vi "QueryWavelength.vi"(8 "error in (no error)":errorcluster, 11 "HRS_Spectrometer in":refnum<class "HRS_Spectrometer.lvclass">) -> (0 "error out":errorcluster, 3 "HRS_Spectrometer out":refnum<class "HRS_Spectrometer.lvclass">)   [LabVIEW 2023, in "HRS_Spectrometer.lvlib" / "HRS_Spectrometer.lvclass"]
uses:
  HRS_Spectrometer.lvclass
  HRS_Spectrometer.lvclass/HRS_Spectrometer.ctl
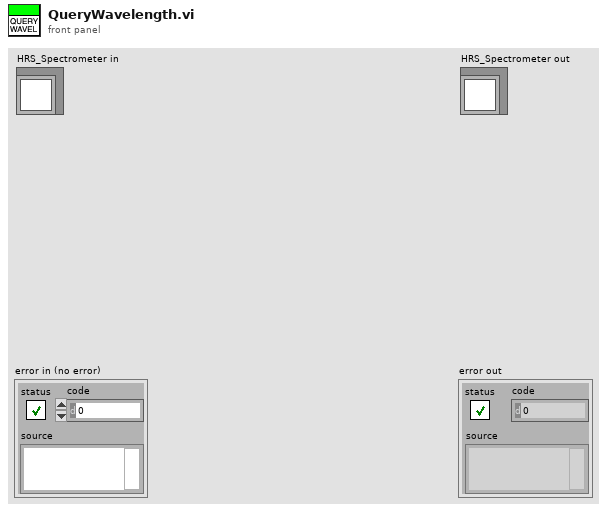
[diagram p1: front panel]
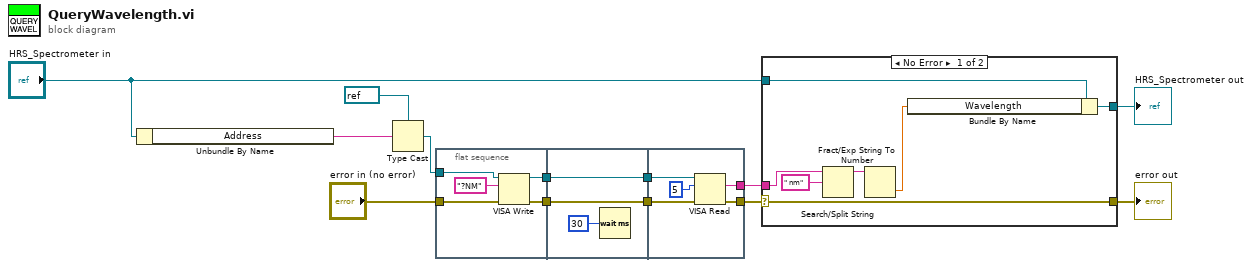
[diagram p0: block diagram]
diagram:
  n1 = Unbundle By Name("HRS_Spectrometer in") -> ("Address"=w1:string)
  n2 = Type Cast(type=refnum<visa-resource-name> refnum ("VISA resource name"), x=w1) -> (*(type *) &x=w2:refnum<visa-resource-name>)
  n3 = flat-sequence {
    tunnel: [w17] -> w13
    tunnel: [w16] -> w12
    tunnel: w2 -> [w15]
    tunnel: "error in (no error)" -> [w14]
    tunnel: w13 -> [w21]
    tunnel: w12 -> [w20]
    tunnel: [w21] -> w11
    tunnel: [w20] -> w10
    tunnel: w11 -> [w25]
    tunnel: w10 -> [w26]
    tunnel: [w24] -> w8
    tunnel: [w23] -> w7
    frame #0 {
      n4 = VISA Write(VISA resource name=w15, write buffer="?NM", error in (no error)=w14) -> (VISA resource name out=w17:refnum<visa-resource-name>, error out=w16:errorcluster)  [unwired: 1 out]
    }
    frame #1 {
      n5 = Wait (ms)(milliseconds to wait=u32 30) -> ()  [unwired: 1 out]
    }
    frame #2 {
      n6 = VISA Read(VISA resource name=w25, byte count=u32 5, error in (no error)=w26) -> (read buffer=w24:string, error out=w23:errorcluster)  [unwired: 2 out]
    }
  }
  n7 = case shown="No Error" w7 {
    selector: w7 -> [w28 w35]
    tunnel: w8 -> [w33 _]
    tunnel: [w30 w34] -> w5
    tunnel: [w28 w35] -> w6
    tunnel: "HRS_Spectrometer in" -> [w27 w34]
    frame No Error {
      n8 = Search/Split String(string=w33, search string/char (-)=" nm") -> (substring before match=w31:string)  [unwired: 1 in, 2 out]
      n9 = Fract/Exp String To Number(string=w31) -> (number=w29:dbl)  [unwired: 3 in, 1 out]
      n10 = Bundle By Name(cluster=w27, "Wavelength"=w29) -> (w30:refnum<class "HRS_Spectrometer.lvclass">)
    }
    frame Error {
    }
  }
  "error out" <- w6
  "HRS_Spectrometer out" <- w5
